vi "Get Temperature.vi"(8 "error in(no error)":errorcluster, 11 "VISA Resource Name":refnum<visa-resource-name>) -> (0 "error out":errorcluster, 2 "temperature [deg C]":dbl, 3 "VISA resource name out":refnum<visa-resource-name>)   [LabVIEW 2018, in "3458A Virtual Digitizer.lvlib" / "3458A Basic Driver.lvlib"]
doc: "Reads temperature of 3458A."
uses:
  3458A Basic Driver.lvlib
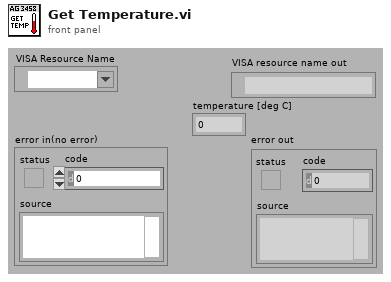
[diagram p1: front panel]
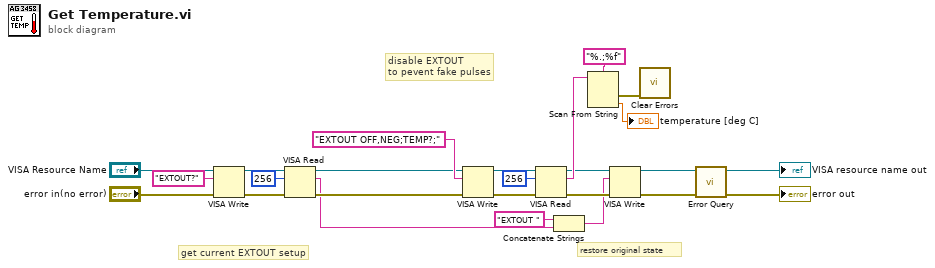
[diagram p0: block diagram]
diagram:
  # "restore original state"
  # "disable EXTOUT\nto pevent fake pulses"
  # "get current EXTOUT setup"
  n1 = VISA Write(VISA resource name="VISA Resource Name", write buffer="EXTOUT?", error in (no error)="error in(no error)") -> (VISA resource name out=w11:refnum<visa-resource-name>, error out=w12:errorcluster)  [unwired: 1 out]
  n2 = VISA Read(VISA resource name=w11, byte count=u32 256, error in (no error)=w12) -> (VISA resource name out=w8:refnum<visa-resource-name>, read buffer=w2:string, error out=w9:errorcluster)  [unwired: 1 out]
  n3 = VISA Write(VISA resource name=w8, write buffer="EXTOUT OFF,NEG;TEMP?;", error in (no error)=w9) -> (VISA resource name out=w23:refnum<visa-resource-name>, error out=w24:errorcluster)  [unwired: 1 out]
  n4 = VISA Read(VISA resource name=w23, byte count=u32 256, error in (no error)=w24) -> (VISA resource name out=w6:refnum<visa-resource-name>, read buffer=w19:string, error out=w7:errorcluster)  [unwired: 1 out]
  n5 = Concatenate Strings("EXTOUT " ("string"), w2) -> (w3:string)
  n6 = Scan From String(format string="%.;%f", input string=w19) -> (error out=w20:errorcluster, output 1=→"temperature [deg C]":dbl)  [unwired: 3 in, 2 out]
  n7 = VISA Write(VISA resource name=w6, write buffer=w3, error in (no error)=w7) -> (VISA resource name out=w5:refnum<visa-resource-name>, error out=w4:errorcluster)  [unwired: 1 out]
  n8 = call <vilib>:"Clear Errors.vi"("error in (no error)"=w20) -> ()  [unwired: 5 in, 2 out]
  n9 = call "Error Query.vi"("error in (no error)"=w4, "VISA resource name"=w5) -> ("error out"=→"error out":errorcluster, "VISA resource name out"=→"VISA resource name out":refnum<visa-resource-name>)  [unwired: 6 in, 2 out]
